vi "QMH Add Message to Queue (Array).vi"(6 "Insert (T)":bool=TRUE, 7 "At Front (F)":bool, 8 "error in (no error)":errorcluster, 9 "Parameters":string[](array[string]), 10 "Messages":string[](array[string]), 11 "queue in":refnum<queue>) -> (0 "error out":errorcluster, 3 "queue out":refnum<queue>)   [LabVIEW 2013, in "QHM.lvlib"]
doc: "Place elements wired to the \"elements\" input on the event queue."
uses:
  QHM.lvlib
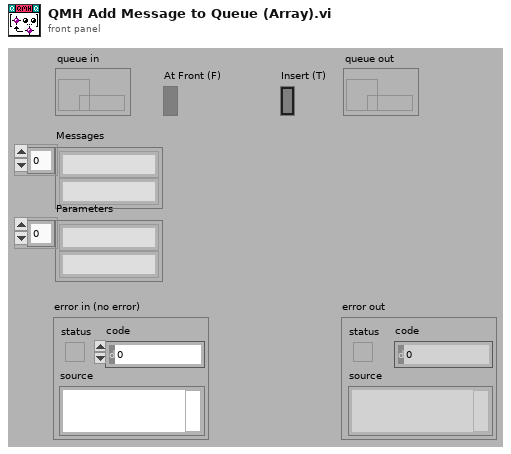
[diagram p1: front panel]
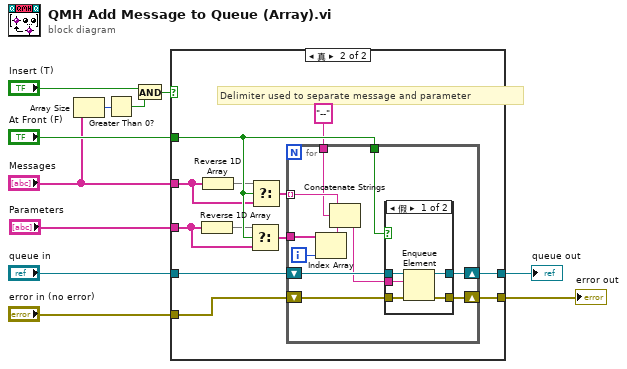
[diagram p0: block diagram]
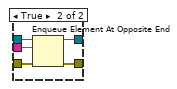
[diagram p3: hidden frame]
diagram:
  n1 = Array Size(array="Messages") -> (size(s)=w3:i32)
  n2 = Greater Than 0?(x=w3) -> (x > 0?=w2:bool)
  n3 = And(x="Insert (T)", y=w2) -> (x .and. y?=w5:bool)
  n4 = case shown="真" w5 {
    tunnel: "error in (no error)" -> [w12 w25]
    tunnel: [w12 w24] -> w10
    tunnel: "queue in" -> [w13 w23]
    tunnel: [w13 w22] -> w8
    tunnel: "At Front (F)" -> [_ w21]
    tunnel: "Messages" -> [_ w20]
    tunnel: "Parameters" -> [_ w19]
    frame False {
    }
    frame True {
      # "Delimiter used to separate message and parameter"
      n5 = Reverse 1D Array(array=w19) -> (reversed array=w16:string[])
      n6 = Reverse 1D Array(array=w20) -> (reversed array=w18:string[])
      n7 = Select(t=w16, s=w21, f=w19) -> (s? t:f=w15:string[])
      n8 = Select(t=w18, s=w21, f=w20) -> (s? t:f=w17:string[])
      n9 = for {
        shift-right: [w34] -> w24
        shift-left: w25 -> [w33]
        tunnel: w17 -> [w31] mode=indexing
        tunnel: w21 -> [w32]
        shift-right: [w35] -> w22
        shift-left: w23 -> [w36]
        tunnel: w15 -> [w28]
        tunnel: "--" ("string") -> [w30]
        i -> [w26]
        n10 = Index Array(array=w28, index=w26) -> (element=w27:string)
        n11 = Concatenate Strings(w31, w30, w27) -> (w29:string)
        n12 = case shown="假" w32 {
          tunnel: w29 -> [w41 w46]
          tunnel: w36 -> [w40 w42]
          tunnel: [w39 w43] -> w35
          tunnel: [w38 w44] -> w34
          tunnel: w33 -> [w37 w45]
          frame False {
            n13 = Enqueue Element(queue=w40, element=w41, error in (no error)=w37) -> (queue out=w39:refnum<queue>, error out=w38:errorcluster)  [unwired: 1 in, 1 out]
          }
          frame True {
            n14 = Enqueue Element At Opposite End(queue=w42, element=w46, error in (no error)=w45) -> (queue out=w43:refnum<queue>, error out=w44:errorcluster)  [unwired: 1 in, 1 out]
          }
        }
      }
    }
  }
  "error out" <- w10
  "queue out" <- w8
